vi "Voltage2Angle.vi"(11 "Voltage":dbl) -> (3 "Angle":dbl)   [LabVIEW 2021]
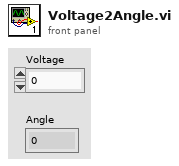
[diagram p1: front panel]
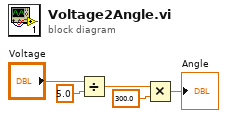
[diagram p0: block diagram]
diagram:
  n1 = Divide(x="Voltage", y=5.0) -> (x/y=w3:dbl)
  n2 = Multiply(x=w3, y=300.0) -> (x*y=→"Angle":dbl)
